vi "stimulate_and_record_async.vi"(3 "SSH password":string, 4 "Transfer and Run Date Folder After Experiment":bool, 5 "SSH user name":string, 6 "Tags":string, 7 "Frames":i32, 8 "Convert Power to Voltage":bool, 9 "voltages/power":dbl[](array[numeric]), 10 "parameters":string[](array[string]), 11 "parameters headers":string[](array[string])) -> ()   [LabVIEW 2014]
uses:
  <vilib>/vision/driver/IMAQdx.llb/IMAQdx Acquisition Mode.ctl
  <vilib>/userdefined/High Color/IMAQdx.ctl
  <vilib>/vision/driver/IMAQdx.llb/IMAQdx Buffer Number Mode.ctl
  <vilib>/Utility/file.llb/Write To Spreadsheet File (DBL).vi
  <vilib>/Utility/file.llb/Write To Spreadsheet File (string).vi
  <vilib>/Utility/file.llb/Read From Spreadsheet File (string).vi
  <vilib>/vision/driver/NI_Vision_Acquisition_Software.lvlib
panel:
  out "Saved Buffer Number":u32
  out "ProcessFrameRate":dbl
  out "# elements in queue":i32
  out "CameraFrameRate":dbl
  out "Camera Buffer Number":u32
  out "Image":T1(plugin-control)
  out "JPEG Quality":dbl
  out "Error":string
  out "Save Directory":path
  in  "stop":bool
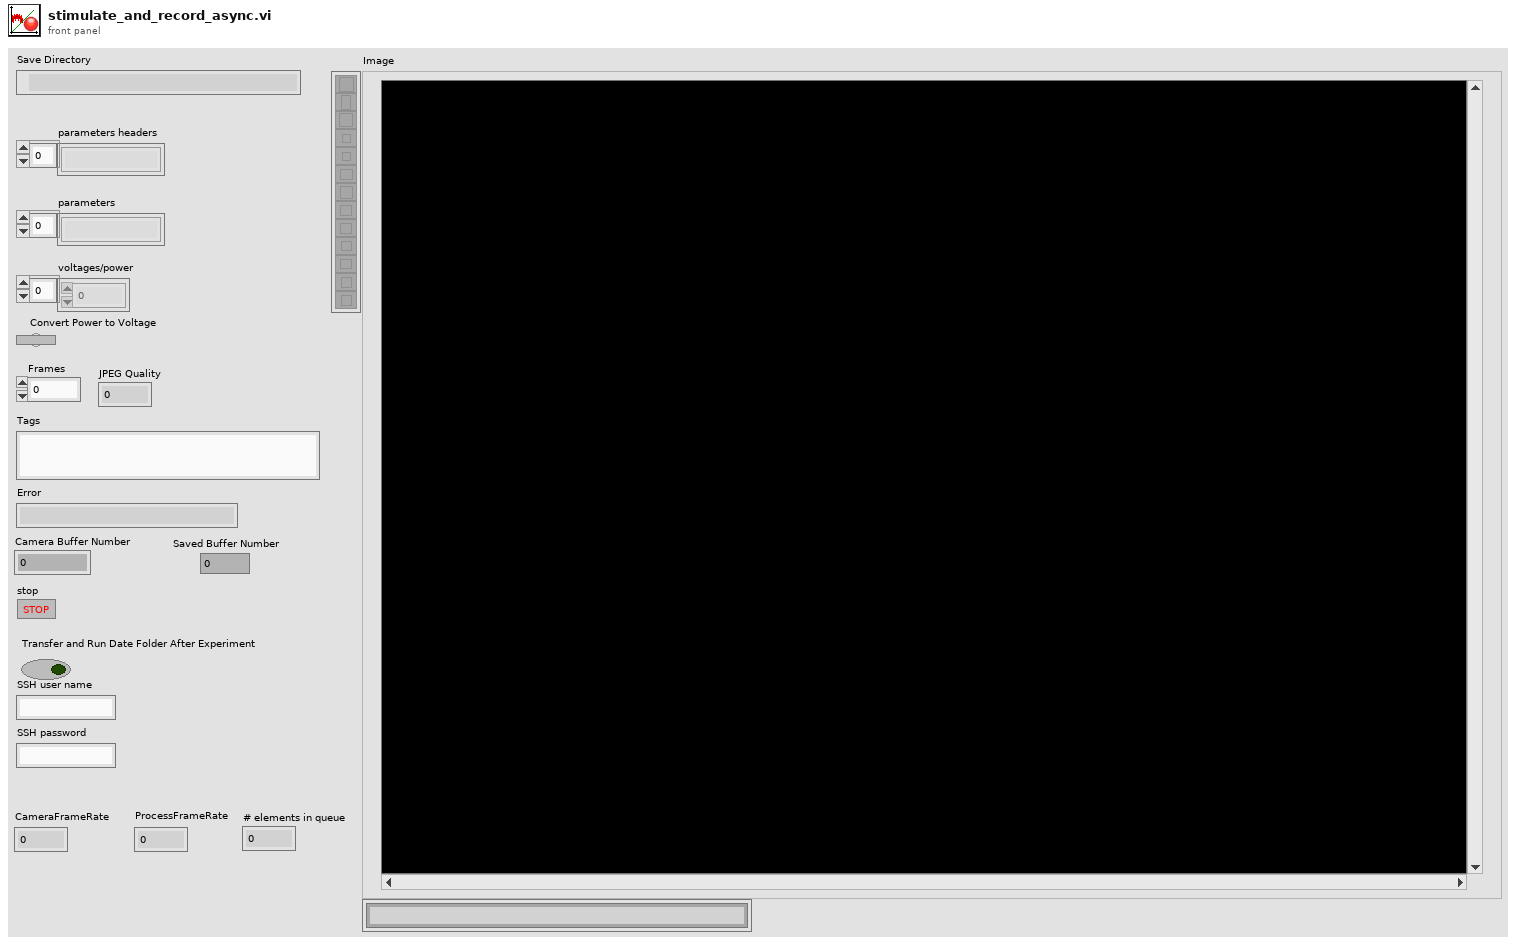
[diagram p1: front panel]
types:
  T1 = typedef "IMAQ Image.ctl" = refnum<image>
  T2 = typedef "IMAQdx.ctl" = refnum<k21>
  T3 = typedef "NI_Vision_Acquisition_Software.lvlib/IMAQdx Buffer Number Mode.ctl" = enum32{"Next", "Last", "Buffer Number"}
  T4 = typedef "Image Type" = u32
  T5 = typedef "NI_Vision_Acquisition_Software.lvlib/IMAQdx Acquisition Mode.ctl" = enum32{"One Shot", "Continuous"}
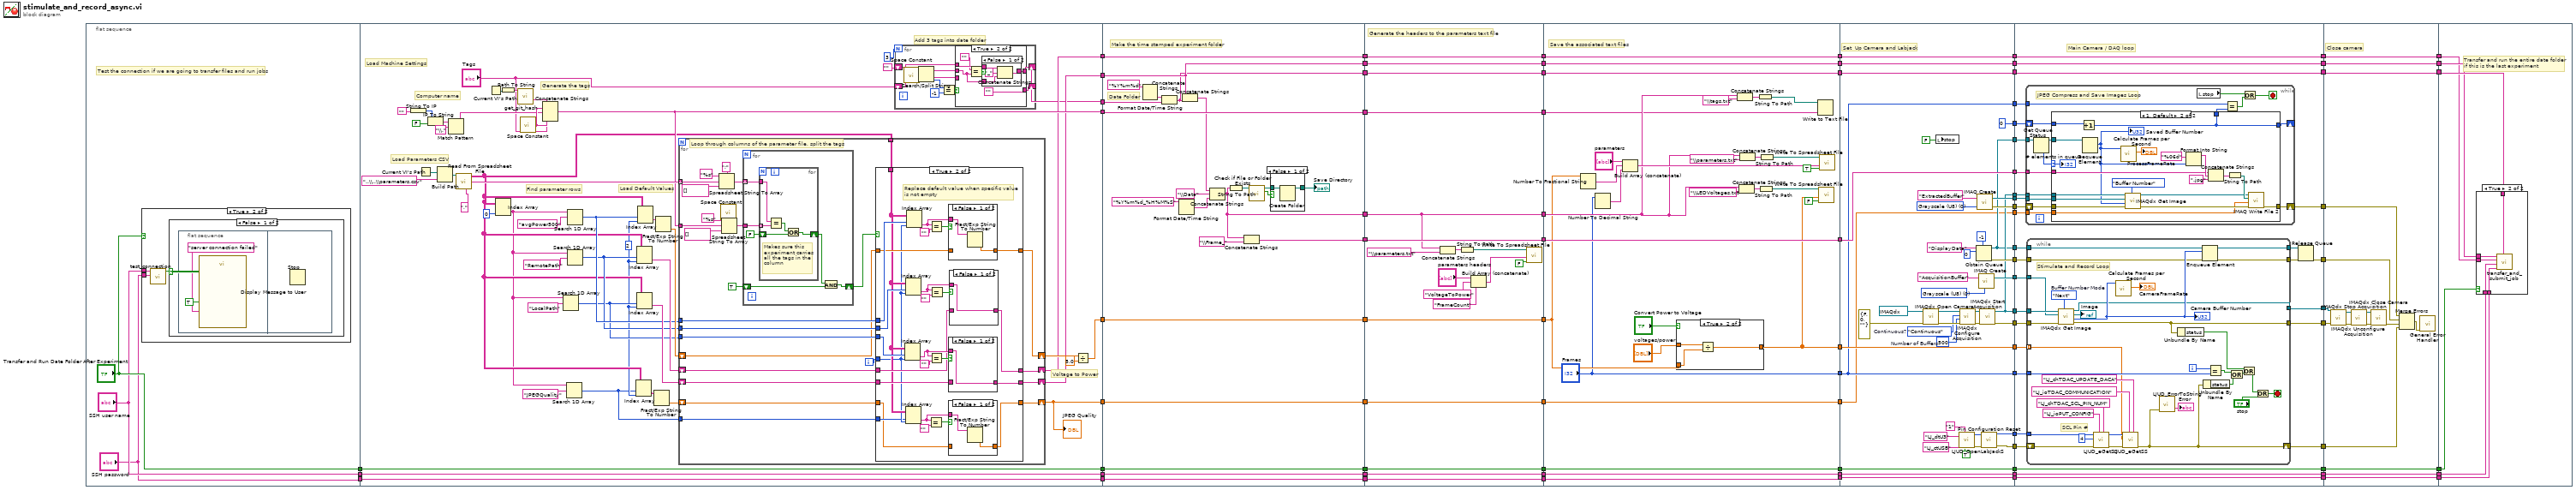
[diagram p0: block diagram]
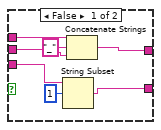
[diagram p4: hidden frame]
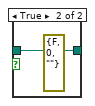
[diagram p11: hidden frame]
diagram:
  n1 = flat-sequence {
    tunnel: ["Transfer and Run Date Folder After Experiment"] -> w47
    tunnel: ["SSH user name"] -> w46
    tunnel: ["SSH password"] -> w45
    tunnel: [w131] -> w77
    tunnel: [w114] -> w76
    tunnel: [w105] -> w67
    tunnel: [w106] -> w66
    tunnel: w47 -> [w123]
    tunnel: w46 -> [w122]
    tunnel: w45 -> [w121]
    tunnel: [w123] -> w38
    tunnel: [w122] -> w31
    tunnel: [w121] -> w30
    tunnel: [w102] -> w23
    tunnel: [w93] -> w22
    tunnel: [w267] -> w61
    tunnel: [w266] -> w59
    tunnel: [w265] -> w57
    tunnel: [w264] -> w55
    tunnel: [w246] -> w53
    tunnel: [w248] -> w51
    tunnel: [w263] -> w49
    tunnel: w66 -> [w263]
    tunnel: w67 -> [w248]
    tunnel: w76 -> [w264]
    tunnel: w77 -> [w265]
    tunnel: [w255] -> w39
    tunnel: w38 -> [w255]
    tunnel: [w254] -> w32
    tunnel: w31 -> [w254]
    tunnel: w30 -> [w253]
    tunnel: [w253] -> w29
    tunnel: w23 -> [w249]
    tunnel: w22 -> [w245]
    tunnel: [w245] -> w19
    tunnel: w61 -> [w289]
    tunnel: [w289] -> w60
    tunnel: w59 -> [w275]
    tunnel: [w275] -> w58
    tunnel: w57 -> [w288]
    tunnel: [w288] -> w56
    tunnel: w55 -> [w287]
    tunnel: [w287] -> w54
    tunnel: w53 -> [w286]
    tunnel: [w286] -> w52
    tunnel: w51 -> [w285]
    tunnel: [w285] -> w50
    tunnel: w49 -> [w284]
    tunnel: [w284] -> w48
    tunnel: [w274] -> w40
    tunnel: w39 -> [w274]
    tunnel: [w273] -> w33
    tunnel: w32 -> [w273]
    tunnel: w29 -> [w272]
    tunnel: [w272] -> w28
    tunnel: [w271] -> w20
    tunnel: w19 -> [w271]
    tunnel: w60 -> [w317]
    tunnel: [w317] -> w82
    tunnel: [w300] -> w80
    tunnel: ["Frames"] -> w79
    tunnel: w58 -> [w309]
    tunnel: w56 -> [w296]
    tunnel: w54 -> [w291]
    tunnel: w52 -> [w305]
    tunnel: [w305] -> w72
    tunnel: [w304] -> w68
    tunnel: w50 -> [w304]
    tunnel: [w303] -> w62
    tunnel: w48 -> [w303]
    tunnel: [w294] -> w41
    tunnel: w40 -> [w294]
    tunnel: [w293] -> w34
    tunnel: w33 -> [w293]
    tunnel: w28 -> [w292]
    tunnel: [w292] -> w27
    tunnel: [w290] -> w21
    tunnel: w20 -> [w290]
    tunnel: w82 -> [w329]
    tunnel: [w359] -> w84
    tunnel: [w358] -> w83
    tunnel: [w362] -> w81
    tunnel: w80 -> [w362]
    tunnel: w79 -> [w328]
    tunnel: [w328] -> w78
    tunnel: [w356] -> w73
    tunnel: w72 -> [w356]
    tunnel: [w355] -> w69
    tunnel: w68 -> [w355]
    tunnel: [w354] -> w63
    tunnel: w62 -> [w354]
    tunnel: [w353] -> w42
    tunnel: w41 -> [w353]
    tunnel: [w352] -> w35
    tunnel: w34 -> [w352]
    tunnel: w27 -> [w351]
    tunnel: [w351] -> w26
    tunnel: w21 -> [w326]
    tunnel: [w335] -> w18
    tunnel: [w330] -> w17
    tunnel: [w334] -> w16
    tunnel: [w333] -> w15
    tunnel: [w327] -> w14
    tunnel: [w332] -> w11
    tunnel: [w331] -> w10
    tunnel: [w330] -> w9
    tunnel: [w329] -> w8
    tunnel: [w328] -> w7
    tunnel: [w327] -> w6
    tunnel: [w326] -> w5
    tunnel: [0] -> w1
    tunnel: w84 -> [w395]
    tunnel: w83 -> [w394]
    tunnel: w81 -> [w393]
    tunnel: w78 -> [w392]
    tunnel: [w391] -> w74
    tunnel: w73 -> [w391]
    tunnel: [w390] -> w70
    tunnel: w69 -> [w390]
    tunnel: [w389] -> w64
    tunnel: w63 -> [w389]
    tunnel: [w388] -> w43
    tunnel: w42 -> [w388]
    tunnel: [w387] -> w36
    tunnel: w35 -> [w387]
    tunnel: w26 -> [w386]
    tunnel: [w386] -> w25
    tunnel: w18 -> [w385]
    tunnel: w17 -> [w384]
    tunnel: w16 -> [w383]
    tunnel: w15 -> [w382]
    tunnel: w14 -> [w381]
    tunnel: [w378] -> w13
    tunnel: [w377] -> w12
    tunnel: w11 -> [w376]
    tunnel: w10 -> [w375]
    tunnel: w9 -> [w374]
    tunnel: w8 -> [w373]
    tunnel: w7 -> [w372]
    tunnel: w6 -> [w371]
    tunnel: w5 -> [w370]
    tunnel: [w369] -> w4
    tunnel: [w368] -> w3
    tunnel: [w367] -> w2
    tunnel: w1 -> [w366]
    tunnel: [w484] -> w75
    tunnel: w74 -> [w484]
    tunnel: [w483] -> w71
    tunnel: w70 -> [w483]
    tunnel: [w482] -> w65
    tunnel: w64 -> [w482]
    tunnel: [w481] -> w44
    tunnel: w43 -> [w481]
    tunnel: [w480] -> w37
    tunnel: w36 -> [w480]
    tunnel: w25 -> [w479]
    tunnel: [w479] -> w24
    tunnel: w13 -> [w474]
    tunnel: w12 -> [w473]
    tunnel: w4 -> [w470]
    tunnel: w3 -> [w469]
    tunnel: w2 -> [w468]
    tunnel: w75 -> [w490]
    tunnel: w71 -> [w489]
    tunnel: w65 -> [w488]
    tunnel: w44 -> [w487]
    tunnel: w37 -> [w486]
    tunnel: w24 -> [w485]
    frame #0 {
      # "Test the connection if we are going to transfer files and run jobs"
      n2 = case shown="True" "Transfer and Run Date Folder After Experiment" {
        tunnel: "SSH password" -> [_ w90]
        tunnel: "SSH user name" -> [_ w88]
        frame False {
        }
        frame True {
          n3 = call "test_connection.vi"("Username"=w88, "Password"=w90) -> ("Connection Successful"=w89:bool)  [unwired: 7 in]
          n4 = case shown="False" w89 {
            frame False {
              n5 = flat-sequence {
                frame #0 {
                  n6 = call "Display Message to User"("Enable"=TRUE, "Message"="server connection failed") -> ()  [unwired: 8 in, 2 out]
                }
                frame #1 {
                  n7 = Stop() -> ()  [unwired: 1 in]
                }
              }
            }
            frame True {
            }
          }
        }
      }
    }
    frame #1 {
      w96 = 2
      # "Add 3 tags into date folder"
      # "Generate the tags"
      # "Find parameter rows"
      # "Load Default Values"
      # "Voltage to Power"
      # "Load Parameters CSV"
      # "Computer name"
      # "Load Machine Settings"
      n8 = String To IP(1:"") -> (0:w139:u32)
      n9 = Current VI's Path() -> (path=w134:path)
      n10 = IP To String(1:FALSE, 2:w139) -> (0:w136:string)
      n11 = Build Path(base path=w134, name or relative path="..\\..\\parameters.csv") -> (appended path=w125:path)
      n12 = Match Pattern(string=w136, regular expression="\\.") -> (before substring=w116:string)  [unwired: 1 in, 3 out]
      n13 = call-poly <vilib>:"Read From Spreadsheet File.vi"("delimiter (\\t)"=",", "file path (dialog if empty)"=w125) -> ("first row"=w115:string[], "all rows"=w98:string[][])  [unwired: 5 in, 3 out]
      n14 = Current VI's Path() -> (path=w118:path)
      n15 = Index Array(array=w98, index (col)=0) -> (element=w97:string[])  [unwired: 1 in]
      n16 = Path To String(path=w118) -> (string=w117:string)
      n17 = call "get_git_hash.vi"("VI folder"=w117) -> ("github hash"=w120:string)  [unwired: 10 in]
      n18 = call <vilib>:"Space Constant.vi"() -> ("String"=w119:string)
      n19 = Concatenate Strings(w120, w119, w116, w119, "Tags") -> (w114:string)
      n20 = Search 1D Array(1D array=w97, element="LocalPath") -> (index of element=w108:i32)  [unwired: 1 in]
      n21 = Search 1D Array(1D array=w97, element="JPEGQuality") -> (index of element=w94:i32)  [unwired: 1 in]
      n22 = Search 1D Array(1D array=w97, element="RemotePath") -> (index of element=w109:i32)  [unwired: 1 in]
      n23 = Search 1D Array(1D array=w97, element="avgPower500") -> (index of element=w110:i32)  [unwired: 1 in]
      n24 = Index Array(array=w98, index (row)=w94, index (col)=w96) -> (element=w99:string)
      n25 = Index Array(array=w98, index (row)=w109, index (col)=w96) -> (element=w112:string)
      n26 = Index Array(array=w98, index (row)=w108, index (col)=w96) -> (element=w111:string)
      n27 = Index Array(array=w98, index (row)=w110, index (col)=w96) -> (element=w127:string)
      n28 = Fract/Exp String To Number(string=w99) -> (number=w95:dbl)  [unwired: 3 in, 1 out]
      n29 = Fract/Exp String To Number(string=w127) -> (number=w113:dbl)  [unwired: 3 in, 1 out]
      n30 = for {
        tunnel: w115 -> [w193] mode=indexing
        tunnel: w114 -> [w185]
        tunnel: w110 -> [w180]
        tunnel: w109 -> [w179]
        tunnel: w108 -> [w178]
        tunnel: w98 -> [w183]
        shift-right: [w175] -> w107
        shift-left: w113 -> [w176]
        shift-right: [w172] -> w106
        shift-left: w112 -> [w173]
        shift-right: [w171] -> w105
        shift-left: w111 -> [w174]
        shift-right: [w168] -> w93
        shift-left: w95 -> [w170]
        tunnel: w94 -> [w169]
        i -> [w177]
        # "Loop through columns of the parameter file, split the tags"
        n31 = Spreadsheet String To Array(delimiter (Tab)=";", format string="%s", spreadsheet string=w193, array type (2D Dbl)=string[] []) -> (array=w189:string[])
        n32 = call <vilib>:"Space Constant.vi"() -> ("String"=w187:string)
        n33 = Spreadsheet String To Array(delimiter (Tab)=w187, format string="%s", spreadsheet string=w185, array type (2D Dbl)=string[] []) -> (array=w184:string[])
        n34 = for {
          tunnel: w189 -> [w239] mode=indexing
          tunnel: w184 -> [w238]
          shift-right: [w236] -> w181
          shift-left: TRUE -> [w234]
          n35 = for {
            tunnel: w239 -> [w244]
            tunnel: w238 -> [w243] mode=indexing
            shift-right: [w240] -> w235
            shift-left: FALSE -> [w241]
            # "Makes sure this\nexperiment carries\nall the tags in the\ncolumn"
            n36 = Equal?(x=w244, y=w243) -> (x = y?=w242:bool)
            n37 = Or(x=w242, y=w241) -> (x .or. y?=w240:bool)
          }
          n38 = And(x=w235, y=w234) -> (x .and. y?=w236:bool)
        }
        n39 = case shown="True" w181 {
          tunnel: w176 -> [w197 w218]
          tunnel: [w197 w217] -> w175
          tunnel: w180 -> [_ w223]
          tunnel: w179 -> [_ w222]
          tunnel: w178 -> [_ w221]
          tunnel: w177 -> [_ w200]
          tunnel: w183 -> [_ w201]
          tunnel: [w196 w207] -> w172
          tunnel: [w195 w209] -> w171
          tunnel: w174 -> [w195 w208]
          tunnel: w173 -> [w196 w206]
          tunnel: w170 -> [w194 w198]
          tunnel: w169 -> [_ w199]
          tunnel: [w194 w202] -> w168
          frame False {
          }
          frame True {
            # "Replace default value when specific value\nis not empty"
            n40 = Index Array(array=w201, index (row)=w221, index (col)=w200) -> (element=w210:string)
            n41 = Index Array(array=w201, index (row)=w222, index (col)=w200) -> (element=w213:string)
            n42 = Index Array(array=w201, index (row)=w199, index (col)=w200) -> (element=w203:string)
            n43 = Index Array(array=w201, index (row)=w223, index (col)=w200) -> (element=w216:string)
            n44 = Equal?(x=w203, y="") -> (x = y?=w204:bool)
            n45 = Equal?(x=w216, y="") -> (x = y?=w219:bool)
            n46 = Equal?(x=w210, y="") -> (x = y?=w211:bool)
            n47 = Equal?(x=w213, y="") -> (x = y?=w214:bool)
            n48 = case shown="False" w204 {
              tunnel: w198 -> [_ w226]
              tunnel: [w225 w226] -> w202
              tunnel: w203 -> [w224 _]
              frame False {
                n49 = Fract/Exp String To Number(string=w224) -> (number=w225:dbl)  [unwired: 3 in, 1 out]
              }
              frame True {
              }
            }
            n50 = case shown="False" w219 {
              tunnel: w218 -> [_ w233]
              tunnel: [w232 w233] -> w217
              tunnel: w216 -> [w231 _]
              frame False {
                n51 = Fract/Exp String To Number(string=w231) -> (number=w232:dbl)  [unwired: 3 in, 1 out]
              }
              frame True {
              }
            }
            n52 = case shown="False" w211 {
              tunnel: w210 -> [w227 _]
              tunnel: [w227 w228] -> w209
              tunnel: w208 -> [_ w228]
              frame False {
              }
              frame True {
              }
            }
            n53 = case shown="False" w214 {
              tunnel: w213 -> [w229 _]
              tunnel: [w229 w230] -> w207
              tunnel: w206 -> [_ w230]
              frame False {
              }
              frame True {
              }
            }
          }
        }
      }
      "JPEG Quality" <- w93
      n54 = for {
        N: 3 -> [_]
        shift-right: [w140] -> _
        shift-left: "Tags" -> [w149]
        shift-right: [w142] -> w102
        shift-left: "" -> [w147]
        n55 = call <vilib>:"Space Constant.vi"() -> ("String"=w148:string)
        n56 = Search/Split String(string=w149, search string/char (-)=w148) -> (substring before match=w146:string, match + rest of string=w145:string, offset of match=w144:i32)  [unwired: 1 in]
        n57 = Equal?(x=w144, y=-1) -> (x = y?=w141:bool)
        n58 = case shown="True" w141 {
          tunnel: w147 -> [w150 w160]
          tunnel: w146 -> [w151 w157]
          tunnel: w145 -> [w152 _]
          tunnel: [w154 ""] -> w140
          tunnel: [w153 w159] -> w142
          frame False {
            n59 = String Subset(string=w152, offset (0)=1) -> (substring=w154:string)  [unwired: 1 in]
            n60 = Concatenate Strings(w150, "_", w151) -> (w153:string)
          }
          frame True {
            n61 = Equal?(x="", y=w157) -> (x = y?=w161:bool)
            n62 = case shown="False" w161 {
              tunnel: w160 -> [w164 w167]
              tunnel: [w165 w167] -> w159
              tunnel: w157 -> [w163 _]
              frame False {
                n63 = Concatenate Strings(w164, "_", w163) -> (w165:string)
              }
              frame True {
              }
            }
          }
        }
      }
      n64 = Divide(x=w107, y=5.0) -> (x/y=w131:dbl)
    }
    frame #2 {
      # "Make the time stamped experiment folder"
      # "Date Folder"
      n65 = Format Date/Time String(time format string (%c)="%Y%m%d") -> (date/time string=w250:string)  [unwired: 2 in]
      n66 = Concatenate Strings(w250, w249) -> (w246:string)
      n67 = Format Date/Time String(time format string (%c)="%Y%m%d_%H%M%S") -> (date/time string=w252:string)  [unwired: 2 in]
      n68 = Concatenate Strings(w248, w246) -> (w247:string)
      n69 = Concatenate Strings(w247, "\\Data", w252) -> (w266:string)
      n70 = String To Path(string=w266) -> (path=w258:path)
      n71 = Concatenate Strings(w266, "\\Frame_") -> (w267:string)
      n72 = call <vilib>:"Check if File or Folder Exists.vi"("path"=w258) -> ("file or folder exists?"=w261:bool, "dup path"=w260:path)  [unwired: 8 in, 1 out]
      n73 = case shown="False" w261 {
        tunnel: [w268 w270] -> w257
        tunnel: w260 -> [w269 w270]
        frame False {
          n74 = Create Folder(path (use dialog)=w269) -> (created path=w268:path)  [unwired: 2 in, 2 out]
        }
        frame True {
          (unwired) errorcluster {"status"=FALSE, "code"=0, "source"=""} ("error out")
        }
      }
      "Save Directory" <- w257
    }
    frame #3 {
      # "Generate the headers to the parameters text file"
      n75 = Concatenate Strings(w275, "\\parameters.txt") -> (w283:string)
      n76 = String To Path(string=w283) -> (path=w282:path)
      n77 = Build Array (concatenate)("parameters headers", "VoltageToPower", "FrameCount") -> (w279:string[])
      n78 = call-poly <vilib>:"Write To Spreadsheet File.vi"("append to file? (new file:F)"=FALSE, "1D data"=w279, "file path (dialog if empty)"=w282) -> ()  [unwired: 5 in, 1 out]
    }
    frame #4 {
      # "Save the associated text files"
      n79 = Number To Fractional String(number=w296) -> (F-format string=w297:string)  [unwired: 3 in]
      n80 = Number To Decimal String(number="Frames") -> (decimal integer string=w298:string)  [unwired: 1 in]
      n81 = Build Array (concatenate)("parameters", w297, w298) -> (w310:string[])
      n82 = case shown="True" "Convert Power to Voltage" {
        tunnel: "voltages/power" -> [w320 w323]
        tunnel: [w320 w321] -> w300
        tunnel: w296 -> [_ w322]
        frame False {
        }
        frame True {
          n83 = Divide(x=w323, y=w322) -> (x/y=w321:dbl[])
        }
      }
      n84 = Concatenate Strings(w309, "\\tags.txt") -> (w307:string)
      n85 = Concatenate Strings(w309, "\\LEDVoltages.txt") -> (w319:string)
      n86 = Concatenate Strings(w309, "\\parameters.txt") -> (w314:string)
      n87 = String To Path(string=w307) -> (path=w306:path)
      n88 = String To Path(string=w319) -> (path=w318:path)
      n89 = String To Path(string=w314) -> (path=w313:path)
      n90 = Write to Text File(file (use dialog)=w306, text=w291) -> ()  [unwired: 2 in, 3 out]
      n91 = call-poly <vilib>:"Write To Spreadsheet File.vi"("append to file? (new file:F)"=FALSE, "1D data"=w300, "file path (dialog if empty)"=w318) -> ()  [unwired: 5 in, 1 out]
      n92 = call-poly <vilib>:"Write To Spreadsheet File.vi"("append to file? (new file:F)"=TRUE, "1D data"=w310, "file path (dialog if empty)"=w313) -> ()  [unwired: 5 in, 1 out]
    }
    frame #5 {
      w338 = T4 0 items=["Grayscale (U8)", "Grayscale (I16)", "Grayscale (SGL)", "Complex (CSG)", "RGB (U32)", "HSL (U32)", "RGB (U64)"] ("Image Type")
      w347 = T4 0 items=["Grayscale (U8)", "Grayscale (I16)", "Grayscale (SGL)", "Complex (CSG)", "RGB (U32)", "HSL (U32)", "RGB (U64)"] ("Image Type")
      w348 = u32 500  # Number of Buffers
      w344 = IMAQdx_Acquisition_Mode."Continuous"  # Continuous?
      # "Set  Up Camera and Labjack"
      n93 = call <vilib>:"IMAQdx Open Camera.vi"("error in"=errorcluster {"status"=FALSE, "code"=0, "source"=""}, "Session In"=T2 "cam0") -> ("error out"=w349:errorcluster, "Session Out"=w350:T2)  [unwired: 8 in]
      n94 = local write "stop"(FALSE) -> ()
      n95 = call "LJUD_OpenLabJackS.vi"("FirstFound"=TRUE, "Address"="1" ("DeviceType"), "ConnectionType"="LJ_ctUSB", "DeviceType"="LJ_dtU3") -> ("error out"=w357:errorcluster, "Handle"=w360:i32)  [unwired: 5 in, 1 out]
      n96 = call <vilib>:"IMAQdx Configure Acquisition.vi"("error in"=w349, "Number of Buffers"=w348, "Continuous?"=w344, "Session In"=w350) -> ("error out"=w345:errorcluster, "Session Out"=w343:T2)  [unwired: 6 in]
      n97 = Obtain Queue(max queue size (-1, unlimited)=-1, name (unnamed)="DisplayData", element data type=u32 0) -> (queue out=w327:refnum<queue>, error out=w333:errorcluster)  [unwired: 2 in, 1 out]
      n98 = call "IMAQ Create"("Image Name"="ExtractedBuffer", "Image Type"=w338) -> ("New Image"=w331:T1, "error out"=w332:errorcluster)  [unwired: 3 in]
      n99 = call "IMAQ Create"("Image Name"="AcquisitionBuffer", "Image Type"=w347) -> ("New Image"=w334:T1)  [unwired: 3 in, 1 out]
      n100 = call <vilib>:"IMAQdx Start Acquisition.vi"("error in"=w345, "Session In"=w343) -> ("error out"=w335:errorcluster, "Session Out"=w330:T2)  [unwired: 8 in]
      n101 = call "Pin Configuration Reset.vi"("error in"=w357, "Handle In"=w360) -> ("error out"=w358:errorcluster, "Handle Out"=w359:i32)  [unwired: 8 in]
    }
    frame #6 {
      # "Main Camera / DAQ loop"
      n102 = while {
        tunnel: w371 -> [w411]
        tunnel: w375 -> [w408]
        tunnel: w374 -> [w407]
        tunnel: w373 -> [w405]
        shift-right: [w404] -> w367
        shift-left: w376 -> [w406]
        tunnel: w372 -> [w397]
        tunnel: w370 -> [w402]
        shift-right: [w399] -> _
        shift-left: w366 -> [w400]
        stop <- w403 stop-if-true
        # "JPEG Compress and Save Images Loop"
        n103 = Get Queue Status(queue=w411) -> (queue out=w409:refnum<queue>, # elements in queue=w410:i32)  [unwired: 2 in, 6 out]
        n104 = case shown="1, Default" w410 {
          selector: w410 -> [_ w432]
          tunnel: w409 -> [_ w430]
          tunnel: w408 -> [_ w429]
          tunnel: w407 -> [_ w428]
          tunnel: w406 -> [w413 w427]
          tunnel: w405 -> [_ w421]
          tunnel: [w413 w417] -> w404
          tunnel: w402 -> [_ w416]
          tunnel: w400 -> [w412 w415]
          tunnel: [w412 w414] -> w399
          tunnel: [w412 w414] -> w398
          frame 0 {
          }
          frame 1, Default {
            n105 = Increment(x=w415) -> (x+1=w414:i32)
            n106 = Dequeue Element(queue=w430) -> (element=w418:u32)  [unwired: 2 in, 3 out]
            "Saved Buffer Number" <- w418
            n107 = call <vilib>:"Calculate Frames per Second.vi"("Buffer Number"=w418) -> ("Processed Frames/s"=→"ProcessFrameRate":dbl)  [unwired: 8 in, 2 out]
            n108 = call <vilib>:"IMAQdx Get Image.vi"("Buffer Number Mode (Next)"=IMAQdx_Buffer_Number_Mode."Buffer Number", "error in"=w427, "Buffer Number In"=w418, "Image In"=w429, "Session In"=w428) -> ("error out"=w419:errorcluster, "Image Out"=w420:T1)  [unwired: 3 in, 2 out]
            n109 = Format Into String(format string="%06d" ("string"), w418) -> (resulting string=w423:string)  [unwired: 2 in, 1 out]
            n110 = Concatenate Strings(w421, w423, ".jpg" ("string")) -> (w425:string)
            n111 = String To Path(string=w425) -> (path=w424:path)
            n112 = call-poly "IMAQ Write File 2"("error in (no error)"=w419, "Image Quality"=w416, "File Path"=w424, "Image"=w420) -> ("error out"=w417:errorcluster)  [unwired: 6 in, 1 out]
            "# elements in queue" <- w432
          }
        }
        n113 = local read "stop"() -> (w401:bool)
        n114 = Equal?(x=w397, y=w398) -> (x = y?=w396:bool)
        n115 = Or(x=w401, y=w396) -> (x .or. y?=w403:bool)
      }
      n116 = while {
        tunnel: w395 -> [w452]
        shift-right: [w453] -> w369
        shift-left: w394 -> [w451]
        tunnel: w393 -> [w450] mode=indexing
        tunnel: w392 -> [w461]
        tunnel: w385 -> [w445]
        tunnel: w384 -> [w444]
        tunnel: w383 -> [w443]
        tunnel: w382 -> [w442]
        tunnel: w381 -> [w441]
        tunnel: [w437] -> w380
        tunnel: [w436] -> w379
        tunnel: [w435] -> w378
        tunnel: [w434] -> w377
        i -> [w462]
        stop <- w467 stop-if-true
        w449 = IMAQdx_Buffer_Number_Mode."Next"  # Buffer Number Mode
        # "Stimulate and Record Loop"
        # "SCL Pin #"
        n117 = call <vilib>:"IMAQdx Get Image.vi"("Buffer Number Mode (Next)"=w449, "error in"=w445, "Image In"=w443, "Session In"=w444) -> ("error out"=w434:errorcluster, "Buffer Number Out"=w446:u32, "Image Out"=→"Image":T1, "Session Out"=w435:T2)  [unwired: 4 in]
        "Camera Buffer Number" <- w446
        n118 = call "LJUD_eGetSS.vi"("Channel"="LJ_chTDAC_SCL_PIN_NUM", "IOType"="LJ_ioPUT_CONFIG", "error in"=w451, "Value Write"=4, "Handle In"=w452) -> ("error out"=w454:errorcluster, "Handle Out"=w457:i32)  [unwired: 4 in, 1 out]
        n119 = call <vilib>:"Calculate Frames per Second.vi"("Buffer Number"=w446) -> ("Processed Frames/s"=→"CameraFrameRate":dbl)  [unwired: 8 in, 2 out]
        n120 = call "LJUD_eGetSS.vi"("Channel"="LJ_chTDAC_UPDATE_DACA", "IOType"="LJ_ioTDAC_COMMUNICATION", "error in"=w454, "Value Write"=w450, "Handle In"=w457) -> ("error out"=w453:errorcluster)  [unwired: 4 in, 2 out]
        n121 = call "LJUD_ErrorToString.vi"("error in"=w453) -> ("String"=→"Error":string)  [unwired: 10 in]
        n122 = Unbundle By Name(w434) -> ("status"=w440:bool)
        n123 = Enqueue Element(queue=w441, element=w446, error in (no error)=w442) -> (queue out=w437:refnum<queue>, error out=w436:errorcluster)  [unwired: 1 in, 1 out]
        n124 = Unbundle By Name(w453) -> ("status"=w464:bool)
        n125 = Equal?(x=w462, y=w461) -> (x = y?=w463:bool)
        n126 = Or(x=w463, y=w464) -> (x .or. y?=w439:bool)
        n127 = Or(x=w440, y=w439) -> (x .or. y?=w438:bool)
        n128 = Or(x=w438, y="stop") -> (x .or. y?=w467:bool)
      }
      n129 = Release Queue(queue=w380, error in (no error)=w379) -> (error out=w368:errorcluster)  [unwired: 1 in, 2 out]
    }
    frame #7 {
      # "Close camera"
      n130 = call <vilib>:"IMAQdx Stop Acquisition.vi"("error in"=w473, "Session In"=w474) -> ("error out"=w475:errorcluster, "Session Out"=w476:T2)  [unwired: 8 in]
      n131 = call <vilib>:"IMAQdx Unconfigure Acquisition.vi"("error in"=w475, "Session In"=w476) -> ("error out"=w478:errorcluster, "Session Out"=w477:T2)  [unwired: 8 in]
      n132 = call <vilib>:"IMAQdx Close Camera.vi"("error in"=w478, "Session In"=w477) -> ("error out"=w471:errorcluster)  [unwired: 9 in]
      n133 = Merge Errors(w468, w469, w471, w470) -> (w472:errorcluster)
      n134 = call <vilib>:"General Error Handler.vi"("error in (no error)"=w472) -> ()  [unwired: 10 in, 5 out]
    }
    frame #8 {
      # "Transfer and run the entire date folder\nif this is the last experiment"
      n135 = case shown="True" w487 {
        tunnel: w490 -> [_ w495]
        tunnel: w489 -> [_ w494]
        tunnel: w488 -> [_ w493]
        tunnel: w486 -> [_ w492]
        tunnel: w485 -> [_ w491]
        frame False {
        }
        frame True {
          n136 = call "transfer_and_submit_job.vi"("Date Folder"=w495, "Password"=w491, "Username"=w492, "Remote Data Directory"=w493, "Local Data Directory"=w494) -> ()  [unwired: 7 in]
        }
      }
    }
  }
